vi "screen for user profile.vi"() -> ()   [LabVIEW 2022 SP3]
uses:
  Users/Labview_User/Downloads/Job Cluster.ctl
panel:
  in  "?":bool
  in  "2D Array":cluster{"Job Name Cluster":T1}[][](array[cluster]) {"Job Name Cluster"."Duration" format="%<%Hh%Mm>t"; "Job Name Cluster"."Steps" format="%_1f"; "Job Name Cluster"."Procedures" format="%_1f"}
  # "|"
  # "Procedures"
  # "Steps"
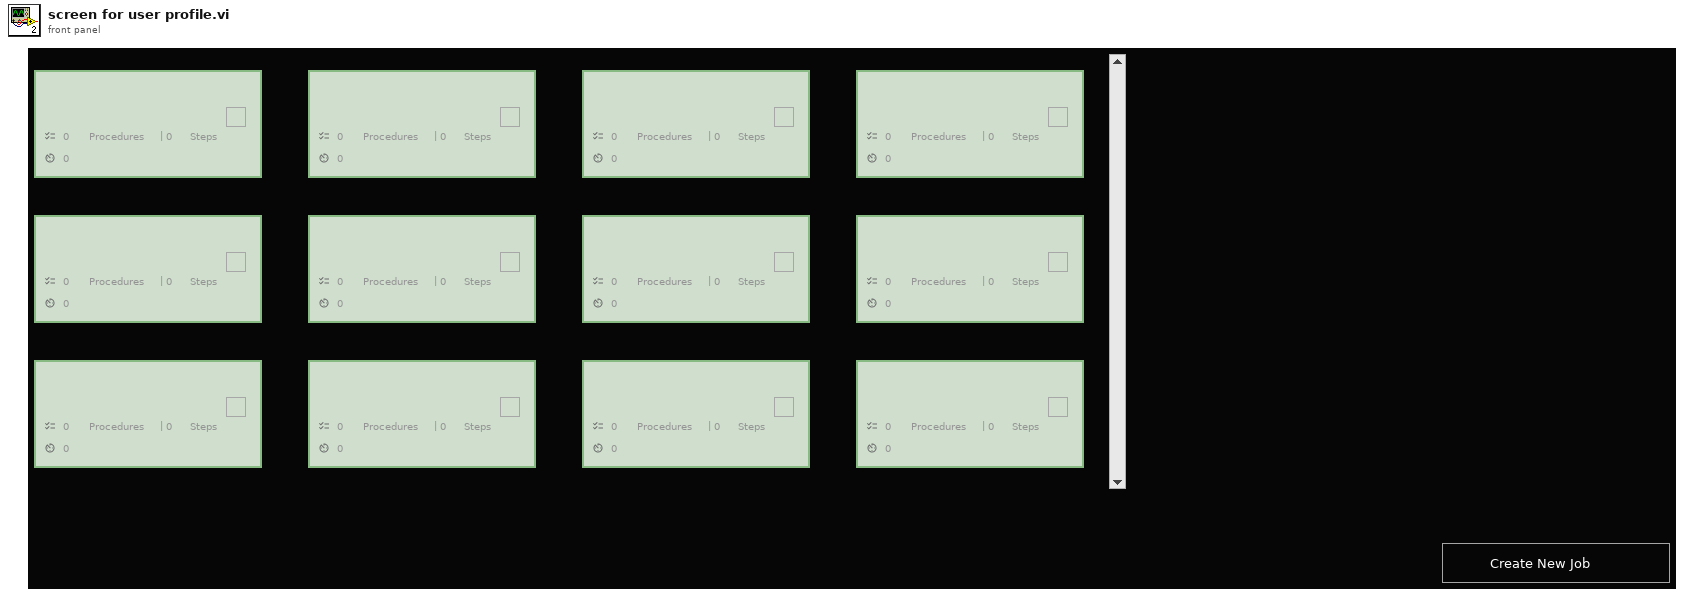
[diagram p1: front panel]
types:
  T1 = typedef "Job Cluster.ctl" = cluster{"Procedures":i32, "Steps":i32, "Duration":i32, "Button":bool, "Job Name":string}
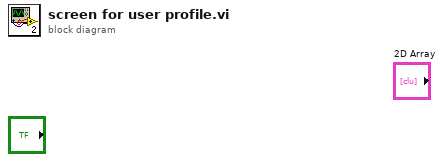
[diagram p0: block diagram]
diagram:
